vi "Close ConvBox.vi"(8 "error in (no error)":errorcluster, 11 "Serial Port":refnum<visa-resource-name>) -> (0 "error out":errorcluster)   [LabVIEW 2023, in "Protocols.lvlib" / "RS-xxx to GPIB ConvBox.lvclass"]
uses:
  RS-xxx to GPIB ConvBox.lvclass
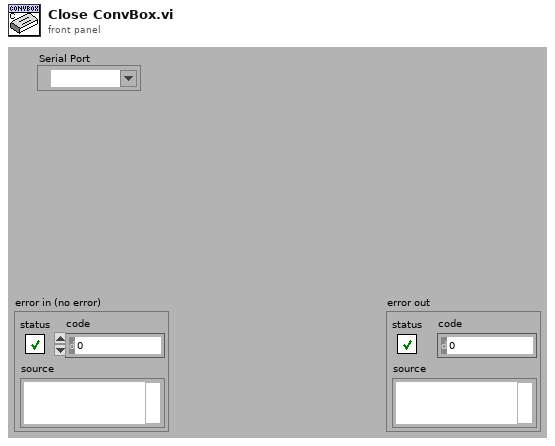
[diagram p1: front panel]
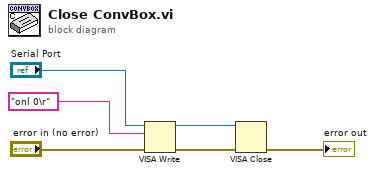
[diagram p0: block diagram]
diagram:
  n1 = VISA Write(VISA resource name="Serial Port", write buffer="onl 0\r", error in (no error)="error in (no error)") -> (VISA resource name out=w3:refnum<visa-resource-name>, error out=w2:errorcluster)  [unwired: 1 out]
  n2 = VISA Close(VISA resource name=w3, error in (no error)=w2) -> (error out=→"error out":errorcluster)
